vi "Bpass.vi"(1 "Input Array":dbl[](array[numeric]) format="%.2f") -> (0 "Output Array":dbl[](array[numeric]) format="%.2f")   [LabVIEW 2011]
uses:
  <vilib>/Analysis/NI_AALBase.lvlib
  <vilib>/Analysis/3filter.llb/Butterworth Filter (DBL).vi
panel:
  out "Error":i32
  in  "Filter Type (def=2)":i32=2
  in  "High Frequency Cutoff":i32=500
  in  "Low Frequency Cutoff":i32=20
  in  "Sampling Frequency":i32=1000
  # "0 = Lowpass\n1 = Highpass\n2 = Bandpass (default)\n3 = Bandstop"
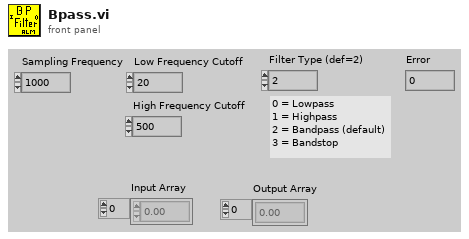
[diagram p1: front panel]
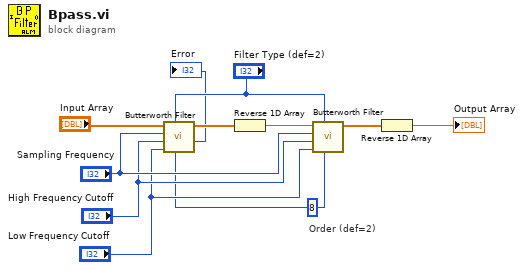
[diagram p0: block diagram]
diagram:
  w2 = 8  # Order (def=2)
  n1 = call-poly <vilib>:"Butterworth Filter.vi"("order"=w2, "filter type"="Filter Type (def=2)", "low cutoff freq: fl"="Low Frequency Cutoff", "high cutoff freq: fh"="High Frequency Cutoff", "sampling freq: fs"="Sampling Frequency", "X"="Input Array") -> ("error"=→"Error":i32, "Filtered X"=w9:dbl[])  [unwired: 2 in]
  n2 = Reverse 1D Array(array=w9) -> (reversed array=w8:dbl[])
  n3 = call-poly <vilib>:"Butterworth Filter.vi"("order"=w2, "filter type"="Filter Type (def=2)", "low cutoff freq: fl"="Low Frequency Cutoff", "high cutoff freq: fh"="High Frequency Cutoff", "sampling freq: fs"="Sampling Frequency", "X"=w8) -> ("Filtered X"=w7:dbl[])  [unwired: 2 in, 1 out]
  n4 = Reverse 1D Array(array=w7) -> (reversed array=→"Output Array":dbl[])
